vi "Read FIFO.vi"(7 "error in (no error)":errorcluster, 9 "Output Values in":dbl[](array[numeric]), 10 "Refnum in":refnum<k33>) -> (0 "error out":errorcluster, 2 "Output Values out":dbl[](array[numeric]), 3 "Refnum out":refnum<k33>)   [LabVIEW 2017, in "Shared Variables CD 2.0 Engine.lvlib"]
uses:
  Shared Variables CD 2.0 Engine.lvlib
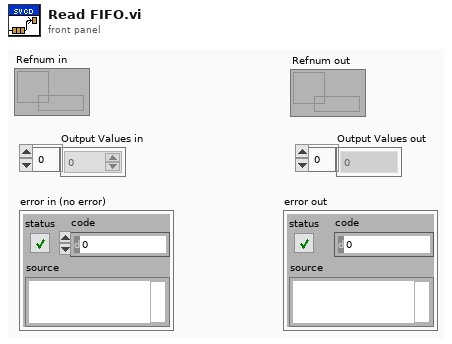
[diagram p1: front panel]
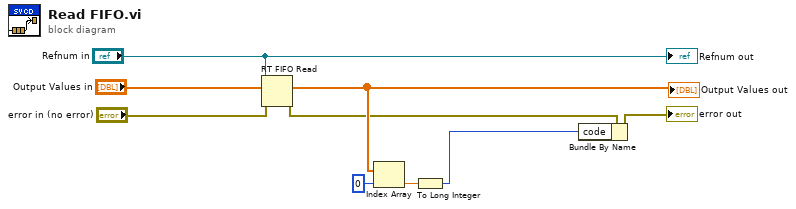
[diagram p0: block diagram]
diagram:
  n1 = RT FIFO Read(0:"Refnum in", 1:"Output Values in", 3:"error in (no error)") -> (9:w5:dbl[], 11:w3:errorcluster)  [unwired: 1 in, 3 out]
  "Output Values out" <- w5
  n2 = Index Array(array=w5, index=0) -> (element=w7:dbl)
  n3 = To Long Integer(number=w7) -> (32bit integer=w9:i32)
  n4 = Bundle By Name(cluster=w3, "code"=w9) -> (→"error out":errorcluster)
  "Refnum out" <- "Refnum in"
